vi "PJT_05.vi"() -> ()   [LabVIEW 2019]
panel:
  out "슬라이드 2":dbl(slide) scale=0.0..10.0
  in  "슬라이드":dbl(slide) scale=0.0..10.0
  out "a-b":dbl
  out "a+b":dbl
  in  "b":dbl
  in  "a":dbl
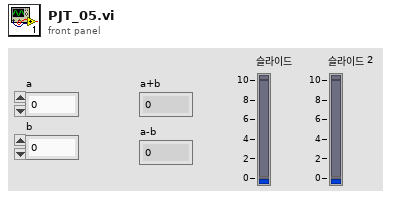
[diagram p1: front panel]
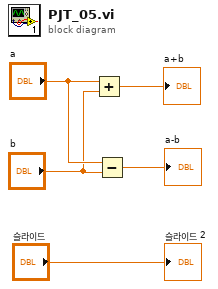
[diagram p0: block diagram]
diagram:
  n1 = Add(x="a", y="b") -> (x+y=→"a+b":dbl)
  n2 = Subtract(x="a", y="b") -> (x-y=→"a-b":dbl)
  "슬라이드 2" <- "슬라이드"
